vi "polyphase_clock_sync.vi"(0 "samples":cdb[](array[numeric]), 5 "nfilts":i32, 7 "sps":i32, 9 "taps":dbl[][](array[numeric]), 11 "diff taps":dbl[][](array[numeric]), 12 "alpha":dbl format="%#_13g", 13 "beta":dbl format="%#_13g") -> (4 "out symbols":cdb[](array[numeric]), 15 "error":dbl[](array[numeric]) format="%#_6p")   [LabVIEW 2014]
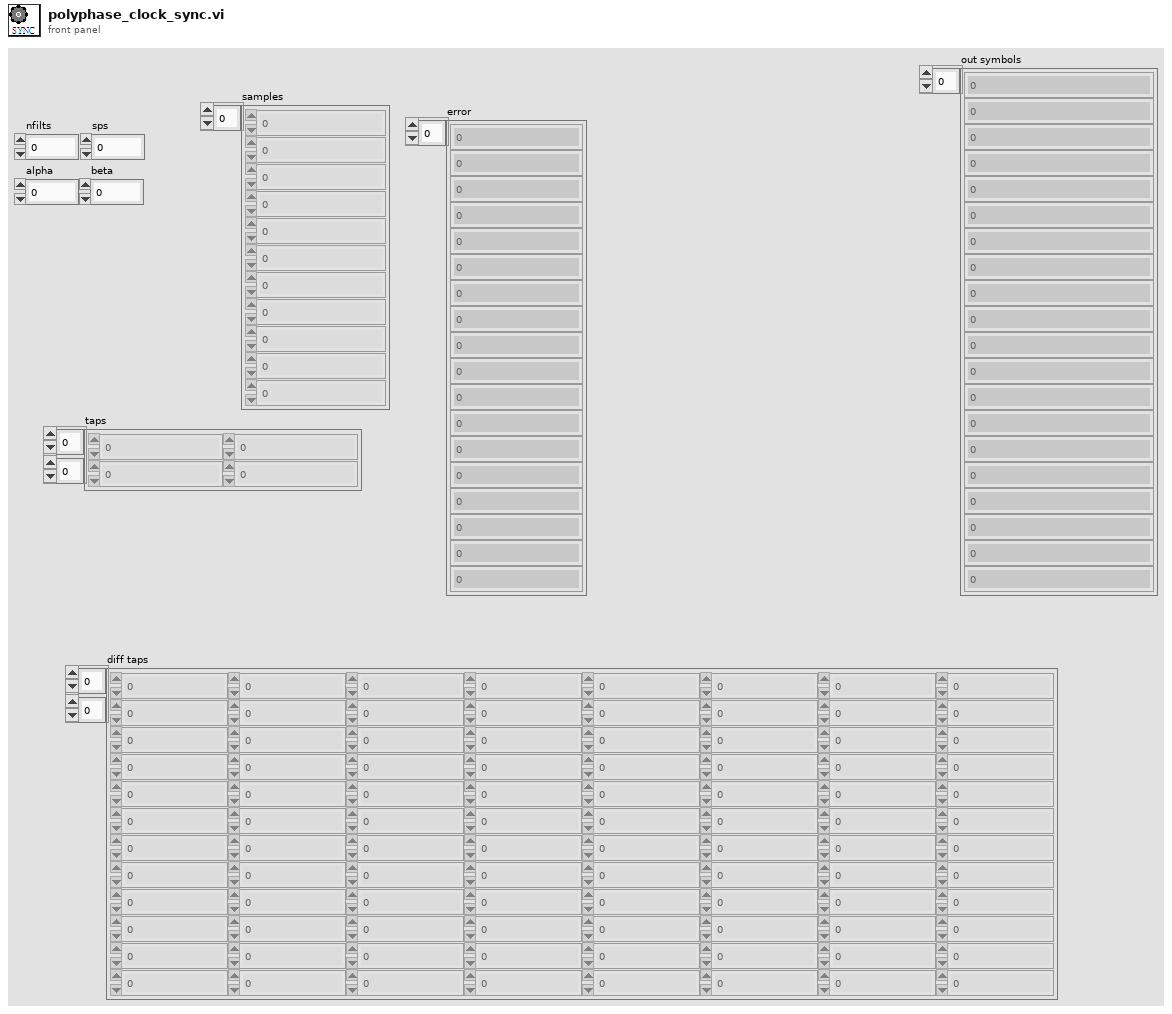
[diagram p1: front panel]
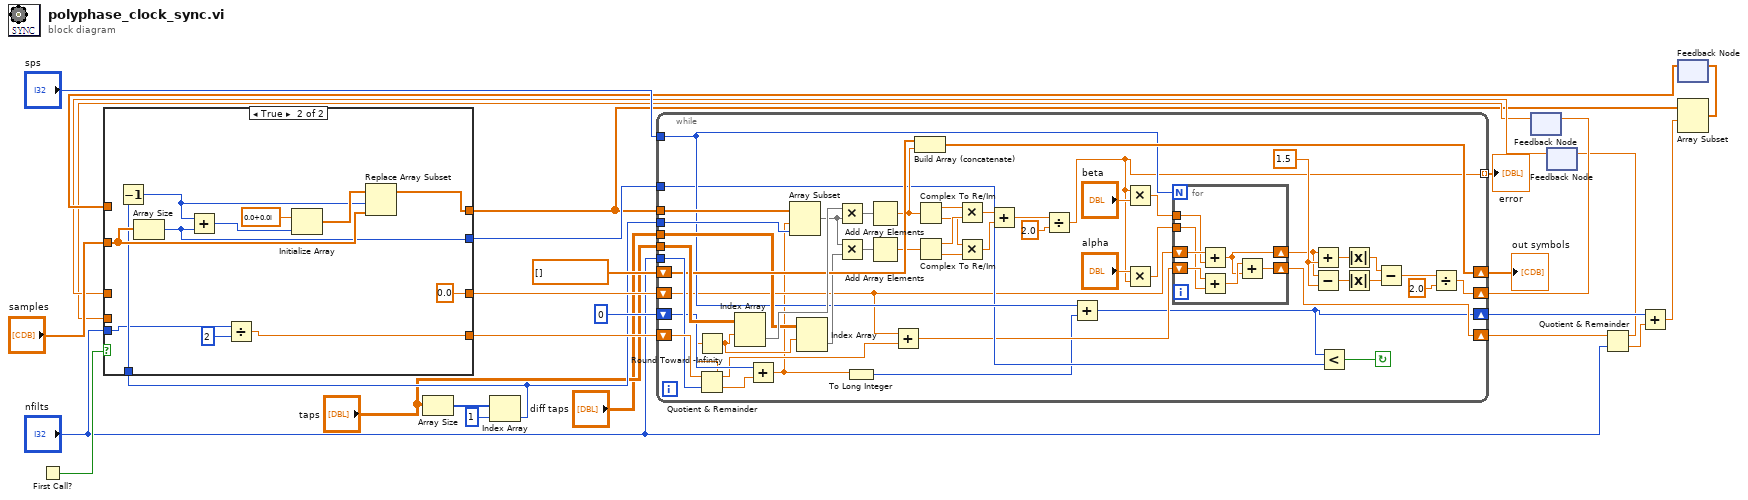
[diagram p0: block diagram]
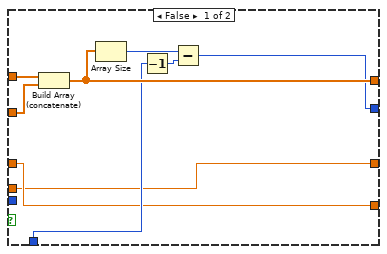
[diagram p2: hidden frame]
diagram:
  n1 = First Call?() -> (First Call?: T/F=w27:bool)
  n2 = Array Size(array="taps") -> (size(s)=w25:i32[])
  n3 = Index Array(array=w25, index=1) -> (element=w7:i32)
  n4 = feedback #1() -> (w14:dbl)  [unwired: 1 in]
  n5 = feedback #2() -> (w16:dbl)  [unwired: 1 in]
  n6 = feedback #3() -> (w17:cdb[])  [unwired: 1 in]
  n7 = case shown="True" w27 {
    tunnel: "nfilts" -> [_ w39]
    tunnel: "samples" -> [w35 w45]
    tunnel: [w34 w44] -> w3
    tunnel: [w31 w43] -> w18
    tunnel: [w28 0.0] -> w23
    tunnel: [w29 w37] -> w22
    tunnel: w17 -> [w36 _]
    tunnel: w16 -> [w29 _]
    tunnel: w14 -> [w28 _]
    tunnel: w7 -> [w30 w41]
    frame False {
      n8 = Build Array (concatenate)(w36, w35) -> (w34:cdb[])
      n9 = Array Size(array=w34) -> (size(s)=w32:i32)
      n10 = Decrement(x=w30) -> (x-1=w33:i32)
      n11 = Subtract(x=w32, y=w33) -> (x-y=w31:i32)
    }
    frame True {
      n12 = Decrement(x=w41) -> (x-1=w40:i32)
      n13 = Array Size(array=w45) -> (size(s)=w43:i32)
      n14 = Add(x=w40, y=w43) -> (x+y=w47:i32)
      n15 = Divide(x=w39, y=2) -> (x/y=w37:dbl)
      n16 = Initialize Array(cdb 0.0+0.0i, w47) -> (w46:cdb[])
      n17 = Replace Array Subset(array=w46, new element=w45, index=w40) -> (w44:cdb[])
    }
  }
  n18 = while {
    tunnel: "taps" -> [w95]
    tunnel: "diff taps" -> [w89]
    tunnel: "nfilts" -> [w97]
    tunnel: "sps" -> [w69]
    tunnel: w3 -> [w93]
    tunnel: w18 -> [w68]
    shift-right: [w57] -> w15
    shift-left: w23 -> [w55]
    shift-right: [w66] -> w6
    shift-left: w22 -> [w98]
    shift-right: [w49] -> w11
    shift-left: 0 -> [w70]
    tunnel: w7 -> [w88]
    shift-right: [w90] -> w19
    shift-left: cdb[] [] -> [w91]
    tunnel: [w56] -> w4 mode=indexing
    stop <- w67 continue-if-true
    w65 = 1.5 ("lim")
    n19 = Quotient & Remainder(x=w98, y=w97) -> (x-y*floor(x/y)=w53:dbl, floor(x/y)=w96:dbl)
    n20 = Round Toward -Infinity(1:w53) -> (0:w52:dbl)
    n21 = Index Array(array=w95, index (row)=w52) -> (element=w94:dbl[])  [unwired: 1 in]
    n22 = Add(x=w70, y=w96) -> (x+y=w51:dbl)
    n23 = Array Subset(array=w93, index=w51, length=w88) -> (w86:cdb[])
    n24 = Index Array(array=w89, index (row)=w52) -> (element=w87:dbl[])  [unwired: 1 in]
    n25 = Multiply(x=w94, y=w86) -> (x*y=w92:cdb[])
    n26 = Multiply(x=w86, y=w87) -> (x*y=w85:cdb[])
    n27 = To Long Integer(number=w51) -> (32bit integer=w50:i32)
    n28 = Add Array Elements(numeric array=w92) -> (sum=w83:cdb)
    n29 = Add Array Elements(numeric array=w85) -> (sum=w84:cdb)
    n30 = Add(x=w55, y=w53) -> (x+y=w54:dbl)
    n31 = Build Array (concatenate)(w91, w83) -> (w90:cdb[])
    n32 = Complex To Re/Im(x + iy=w83) -> (x=w82:dbl, y=w79:dbl)
    n33 = Complex To Re/Im(x + iy=w84) -> (x=w81:dbl, y=w80:dbl)
    n34 = Multiply(x=w82, y=w81) -> (x*y=w77:dbl)
    n35 = Multiply(x=w79, y=w80) -> (x*y=w78:dbl)
    n36 = Add(x=w77, y=w78) -> (x+y=w76:dbl)
    n37 = Divide(x=w76, y=2.0) -> (x/y=w56:dbl)
    n38 = Add(x=w69, y=w50) -> (x+y=w49:i32)
    n39 = Multiply(x=w56, y="beta") -> (x*y=w72:dbl)
    n40 = Multiply(x="alpha", y=w56) -> (x*y=w71:dbl)
    n41 = for {
      N: w69 -> [_]
      shift-right: [w99] -> w66
      shift-left: w54 -> [w103]
      shift-right: [w100] -> w58
      shift-left: w55 -> [w105]
      tunnel: w72 -> [w104]
      tunnel: w71 -> [w102]
      n42 = Add(x=w105, y=w104) -> (x+y=w100:dbl)
      n43 = Add(x=w103, y=w102) -> (x+y=w101:dbl)
      n44 = Add(x=w101, y=w100) -> (x+y=w99:dbl)
    }
    n45 = Add(x=w58, y=w65) -> (x+y=w63:dbl)
    n46 = Subtract(x=w58, y=w65) -> (x-y=w64:dbl)
    n47 = Less?(x=w49, y=w68) -> (x < y?=w67:bool)
    n48 = Absolute Value(x=w63) -> (abs(x)=w62:dbl)
    n49 = Absolute Value(x=w64) -> (abs(x)=w61:dbl)
    n50 = Subtract(x=w62, y=w61) -> (x-y=w60:dbl)
    n51 = Divide(x=w60, y=2.0) -> (x/y=w57:dbl)
  }
  "out symbols" <- w19
  "error" <- w4
  n52 = feedback-in #1(w15) -> ()
  n53 = Quotient & Remainder(x=w6, y="nfilts") -> (x-y*floor(x/y)=w5:dbl, floor(x/y)=w12:dbl)
  n54 = feedback-in #2(w5) -> ()
  n55 = Add(x=w11, y=w12) -> (x+y=w10:dbl)
  n56 = Array Subset(array=w3, index=w10) -> (w9:cdb[])  [unwired: 1 in]
  n57 = feedback-in #3(w9) -> ()
